vi "Read Waveform.vi"   [LabVIEW 2020, in "NH Research Regenerative Test Series.lvlib"]
doc: "Initiates a measurement and returns a waveform containing the instantaneous input voltage or current for the specified phase.\n\nWaveforms are captured with every initiated measurement based on the Set Aperture Length.vi and Set Number of Samples.vi commands."
uses:
  NH Research Regenerative Test Series.lvlib
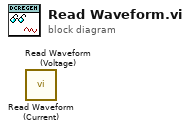
[diagram p0: block diagram]
diagram:
  n1 = call "Read Waveform (Current).vi"() -> ()  [unwired: 13 in, 3 out]
  n2 = call "Read Waveform (Voltage).vi"() -> ()  [unwired: 13 in, 3 out]
